vi "Stacked Shift Registers.vi"() -> ()   [LabVIEW 2015]
panel:
  out "Waveform Chart":cluster{"Scalar":dbl, dbl}(graph)
  in  "stop":bool
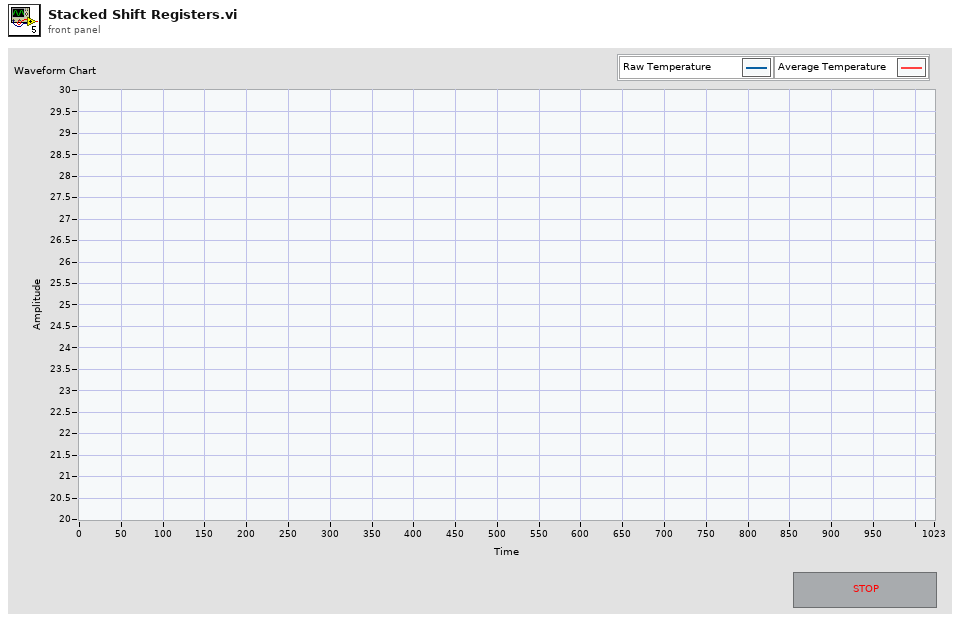
[diagram p1: front panel]
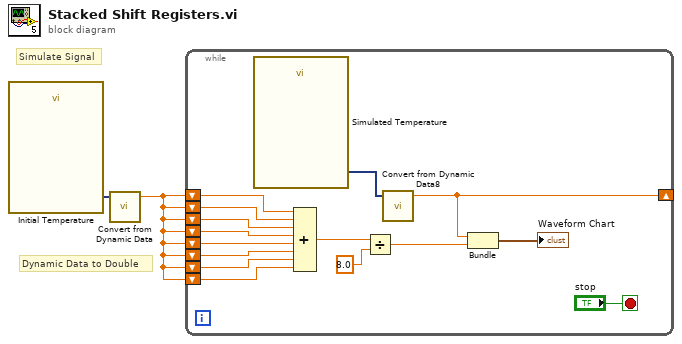
[diagram p0: block diagram]
diagram:
  # "Dynamic Data to Double"
  # "Simulate Signal"
  n1 = call "Initial Temperature"() -> ("Simulated Temperature"=w2:dynamicdata)  [unwired: 14 in, 1 out]
  n2 = call "Convert from Dynamic Data"("Dynamic Data Type"=w2) -> ("Scalar"=w1:dbl)  [unwired: 3 in]
  n3 = while {
    shift-right: [w5] -> _
    shift-left: w1 -> [w15]
    shift-left: w1 -> [w14]
    shift-left: w1 -> [w12]
    shift-left: w1 -> [w11]
    shift-left: w1 -> [w10]
    shift-left: w1 -> [w9]
    shift-left: w1 -> [w8]
    shift-left: w1 -> [w7]
    stop <- "stop" stop-if-true
    n4 = call "Simulated Temperature"() -> ("Simulated Temperature"=w16:dynamicdata)  [unwired: 14 in, 1 out]
    n5 = Compound Arithmetic op=ADD(w15, w14, w12, w11, w10, w9, w8, w7) -> (w13:dbl)
    n6 = Divide(x=w13, y=8.0) -> (x/y=w4:dbl)
    n7 = call "Convert from Dynamic Data8"("Dynamic Data Type"=w16) -> ("Scalar"=w5:dbl)  [unwired: 3 in]
    n8 = Bundle "Bundle"("Scalar"=w5, w4) -> (→"Waveform Chart":cluster{"Scalar":dbl, dbl})  [unwired: 1 in]
  }
